vi "LWXPS_PositionerCorrectorPIDFFAccelerationSet.vi"(0 "Integral gain":dbl, 1 "Derivative gain":dbl, 2 "Integral saturation value":dbl, 3 "Integration time":dbl, 4 "Derivative filter cut off frequency":dbl, 5 "Proportional gain multiplier":dbl, 6 "Integral gain multiplier":dbl, 7 "Derivative gain multiplier":dbl, 8 "Proportional gain":dbl, 9 "Form coefficient":dbl, 10 "Closed Loop Status":bool, 11 "Feed forward acceleration":dbl, 12 "Positioner Name":string, 13 "Feed forward jerk":dbl, 14 "XPS Reference IN":refnum<k24>, 15 "LabVIEW error IN":errorcluster) -> (20 "XPS Reference OUT":refnum<k24>, 22 "Returned error code":i32, 25 "XPS Error String":string, 27 "LabVIEW error OUT":errorcluster)   [LabVIEW 2014]
uses:
  D:/XPSQ8_LabView_Library/Development/Source/Dll/Newport.XPS.CommandInterface.dll
  Dll/Newport.XPS.CommandInterface.dll
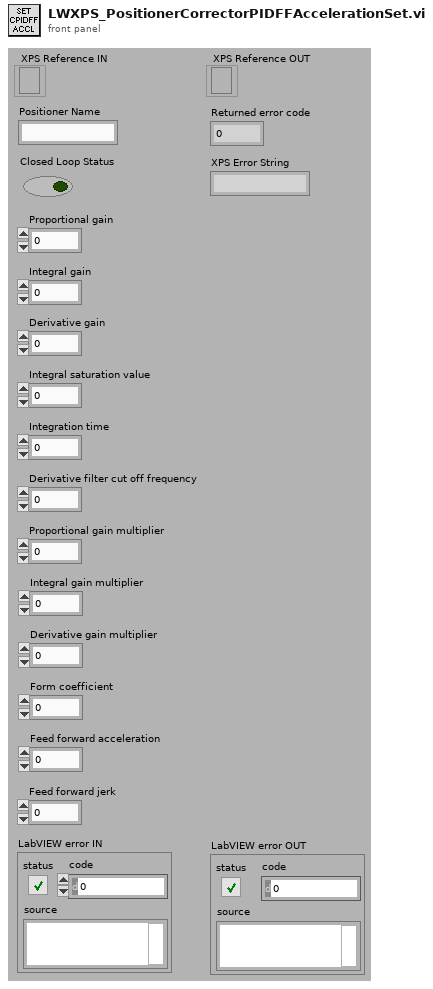
[diagram p1: front panel]
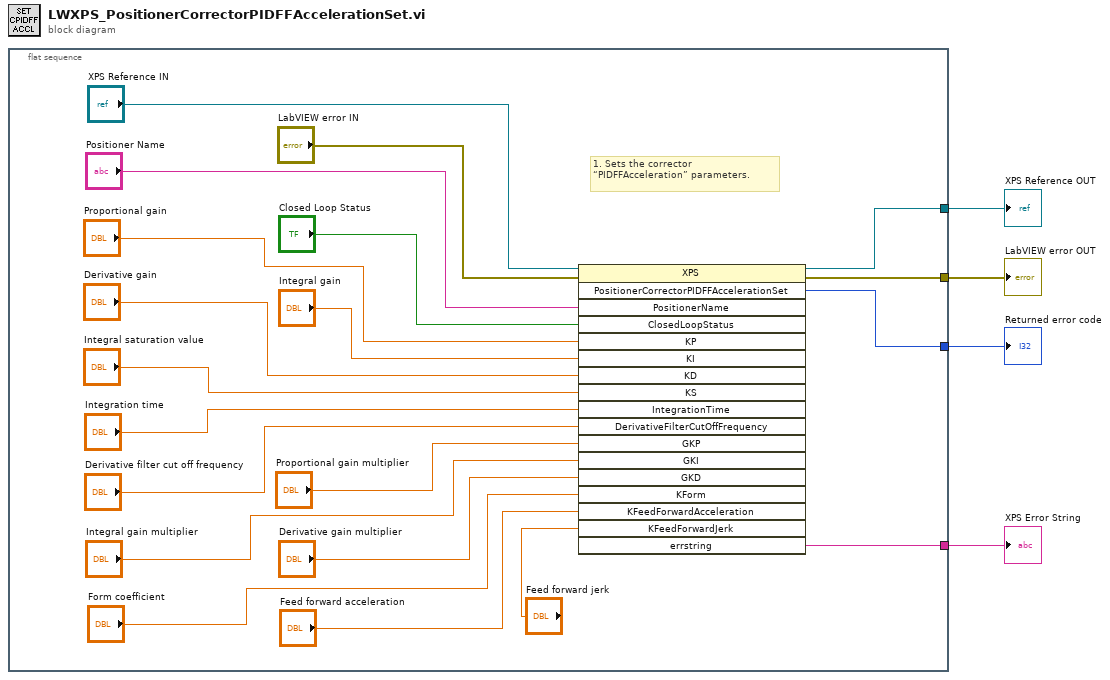
[diagram p0: block diagram]
diagram:
  n1 = flat-sequence {
    tunnel: [w8] -> w4
    tunnel: [w23] -> w3
    tunnel: [w22] -> w2
    tunnel: [w9] -> w1
    frame #0 {
      # "1. Sets the corrector “PIDFFAcceleration” parameters."
      n2 = invoke class="XPS" method="PositionerCorrectorPIDFFAccelerationSet"(reference="XPS Reference IN", error in="LabVIEW error IN", "PositionerName"="Positioner Name", "ClosedLoopStatus"="Closed Loop Status", "KP"="Proportional gain", "KI"="Integral gain", "KD"="Derivative gain", "KS"="Integral saturation value", "IntegrationTime"="Integration time", "DerivativeFilterCutOffFrequency"="Derivative filter cut off frequency", "GKP"="Proportional gain multiplier", "GKI"="Integral gain multiplier", "GKD"="Derivative gain multiplier", "KForm"="Form coefficient", "KFeedForwardAcceleration"="Feed forward acceleration", "KFeedForwardJerk"="Feed forward jerk") -> (reference out=w8:refnum<k24>, error out=w23:errorcluster, "PositionerCorrectorPIDFFAccelerationSet"=w22:i32, "errstring"=w9:string)  [unwired: 2 in, 14 out]
    }
  }
  "XPS Error String" <- w1
  "XPS Reference OUT" <- w4
  "LabVIEW error OUT" <- w3
  "Returned error code" <- w2
